vi "Execute.LoadSequences.vi"(8 "error in (no error)":errorcluster, 11 "Cluster":T1) -> (0 "error out":errorcluster)   [LabVIEW 2013, in "Simple Sequence Editor.lvlib"]
uses:
  Simple Sequence Editor.lvlib
  Types/Execuction.StateVariables.ctl
  Program Files/National Instruments/LabVIEW 2013/examples/NI Veristand/API/Execution API/Sequences/Stimulus Profile Control Tool/Project Execution State.ctl
  <vilib>/NI Veristand/Execution/DataLogging/DataLoggingSpecification Ref.ctl
  NationalInstruments.VeriStand.ClientAPI
  <vilib>/NI Veristand/Execution/DataLogging/IDataLogging Ref.ctl
  <vilib>/NI Veristand/Execution/Workspace/WorkspaceAPI.ctl
  NationalInstruments.VeriStand.RealTimeSequenceDefinitionApi
  Types/Execute.UserEventRefs.ctl
  <vilib>/NI Veristand/Execution/Workspace/SystemStateRegEventRef.ctl
  <vilib>/NI Veristand/Execution/Workspace/SystemStateEventRef.ctl
  NationalInstruments.VeriStand.Internal
  <vilib>/NI Veristand/Execution/Workspace/NI_VS Workspace ExecutionAPI.lvlib
  <vilib>/NI Veristand/Execution/DataLogging/NI_VS Data Logging API.lvlib
panel:
  out "Channels":string[](array[string])
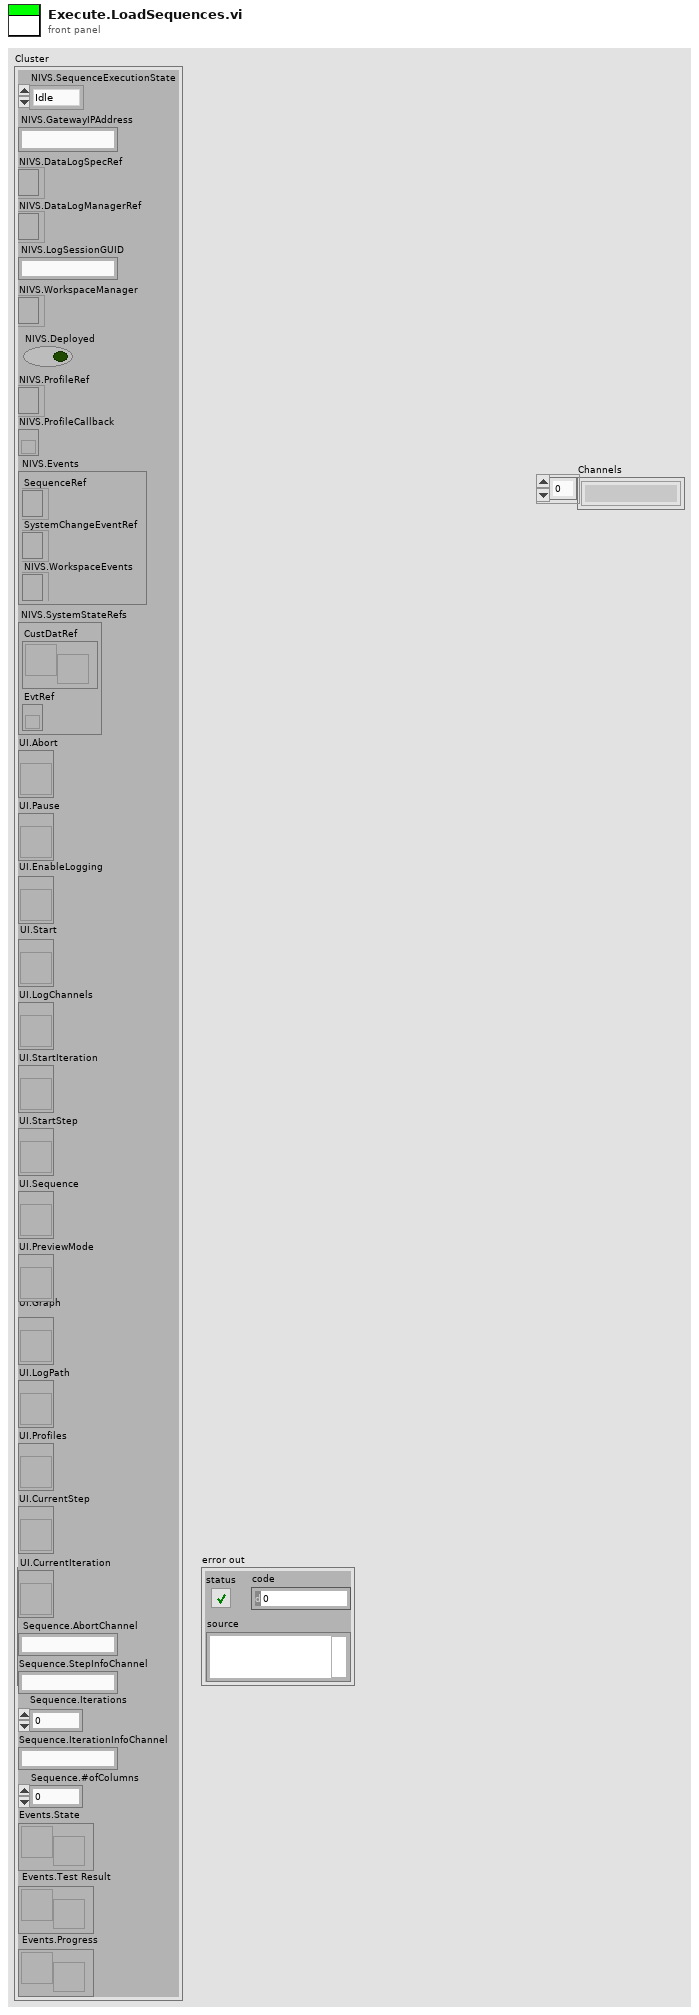
[diagram p1: front panel]
types:
  T1 = typedef "Simple Sequence Editor.lvlib/Execuction.StateVariables.ctl" = cluster{"NIVS.SequenceExecutionState":T2, "NIVS.GatewayIPAddress":string, "NIVS.DataLogSpecRef":T3, "NIVS.DataLogManagerRef":T4, "NIVS.LogSessionGUID":string, "NIVS.WorkspaceManager":T5, "NIVS.Deployed":bool, "NIVS.ProfileRef":refnum<k24>, "NIVS.ProfileCallback":refnum<k27>, "NIVS.Events":T6, "NIVS.SystemStateRefs":T8, "UI.Abort":refnum<vi>, "UI.Pause":refnum<vi>, "UI.EnableLogging":refnum<vi>, "UI.Start":refnum<vi>, "UI.LogChannels":refnum<vi>, "UI.StartIteration":refnum<vi>, "UI.StartStep":refnum<vi>, "UI.Sequence":refnum<vi>, "UI.PreviewMode":refnum<vi>, "UI.Graph":refnum<vi>, "UI.LogPath":refnum<vi>, "UI.Profiles":refnum<vi>, "UI.CurrentStep":refnum<vi>, "UI.CurrentIteration":refnum<vi>, "Sequence.AbortChannel":string, "Sequence.StepInfoChannel":string, "Sequence.Iterations":u32, "Sequence.IterationInfoChannel":string, "Sequence.#ofColumns":i32, "Events.State":refnum<user-event>, "Events.Test Result":refnum<user-event>, "Events.Progress":refnum<user-event>}
  T2 = typedef "Project Execution State.ctl" = enum16{"Idle", "Initializing", "Running", "Paused", "Finalizing", "Complete"}
  T3 = typedef "NI_VS Data Logging API.lvlib/DataLoggingSpecification Ref.ctl" = refnum<k24>
  T4 = typedef "NI_VS Data Logging API.lvlib/IDataLogging Ref.ctl" = refnum<k24>
  T5 = typedef "NI_VS Workspace ExecutionAPI.lvlib/WorkspaceAPI.ctl" = refnum<k24>
  T6 = typedef "Execute.UserEventRefs.ctl" = cluster{"SequenceRef":refnum<event-registration>, "SystemChangeEventRef":T7, "NIVS.WorkspaceEvents":refnum<event-registration>}
  T7 = typedef "NI_VS Workspace ExecutionAPI.lvlib/SystemStateRegEventRef.ctl" = refnum<event-registration>
  T8 = typedef "NI_VS Workspace ExecutionAPI.lvlib/SystemStateEventRef.ctl" = cluster{"CustDatRef":refnum<user-event>, "EvtRef":refnum<k27>}
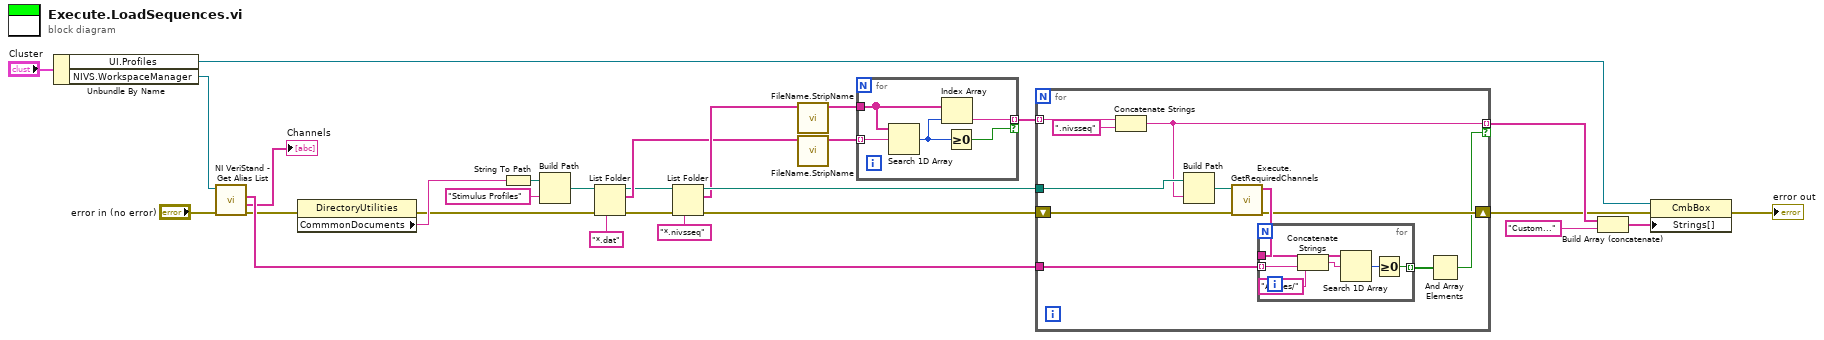
[diagram p0: block diagram]
diagram:
  n1 = Unbundle By Name("Cluster") -> ("UI.Profiles"=w23:refnum<vi>, "NIVS.WorkspaceManager"=w20:T5)
  n2 = call <vilib>:"NI VeriStand - Get Alias List.vi"("error in (no error)"="error in (no error)", "WorkspaceManager in"=w20) -> ("error out"=w4:errorcluster, "Channels"=→"Channels":string[], "Aliases"=w19:string[])  [unwired: 6 in, 1 out]
  n3 = property class="DirectoryUtilities"(error in=w4) -> (error out=w3:errorcluster, "CommmonDocuments"=w6:string)  [unwired: 1 in, 1 out]
  n4 = String To Path(string=w6) -> (path=w7:path)
  n5 = Build Path(base path=w7, name or relative path="Stimulus Profiles") -> (appended path=w2:path)
  n6 = List Folder(path=w2, pattern="*.dat", error in=w3) -> (path out=w8:path, filenames=w11:string[], error out=w16:errorcluster)  [unwired: 1 in, 1 out]
  n7 = List Folder(path=w8, pattern="*.nivsseq", error in=w16) -> (path out=w17:path, filenames=w13:string[], error out=w18:errorcluster)  [unwired: 1 in, 1 out]
  n8 = call "FileName.StripName.vi"("filenames"=w13) -> ("Array"=w14:string[])  [unwired: 10 in]
  n9 = call "FileName.StripName.vi"("filenames"=w11) -> ("Array"=w12:string[])  [unwired: 10 in]
  n10 = for {
    tunnel: w12 -> [w33] mode=indexing
    tunnel: w14 -> [w32]
    tunnel: [w30] -> w15 mode=indexing if=w29
    n11 = Search 1D Array(1D array=w32, element=w33) -> (index of element=w31:i32)  [unwired: 1 in]
    n12 = Index Array(array=w32, index=w31) -> (element=w30:string)
    n13 = Greater Or Equal To 0?(x=w31) -> (x >= 0?=w29:bool)
  }
  n14 = for {
    tunnel: w15 -> [w44] mode=indexing
    tunnel: w17 -> [w42]
    shift-right: [w36] -> w22
    shift-left: w18 -> [w41]
    tunnel: w19 -> [w38]
    tunnel: [w35] -> w24 mode=indexing if=w34
    n15 = Concatenate Strings(w44, ".nivsseq" ("pattern")) -> (w35:string)
    n16 = Build Path(base path=w42, name or relative path=w35) -> (appended path=w40:path)
    n17 = call "Execute.GetRequiredChannels.vi"("error in (no error)"=w41, "Path"=w40) -> ("error out"=w36:errorcluster, "Channels"=w39:string[])  [unwired: 8 in]
    n18 = for {
      tunnel: w39 -> [w50]
      tunnel: w38 -> [w49] mode=indexing
      tunnel: [w47] -> w37 mode=indexing
      n19 = Concatenate Strings("Aliases/", w49) -> (w46:string)
      n20 = Search 1D Array(1D array=w50, element=w46) -> (index of element=w48:i32)  [unwired: 1 in]
      n21 = Greater Or Equal To 0?(x=w48) -> (x >= 0?=w47:bool)
    }
    n22 = And Array Elements(Boolean array=w37) -> (logical AND=w34:bool)
  }
  n23 = Build Array (concatenate)(w24, "Custom...") -> (w25:string[])
  n24 = property class="CmbBox"(reference=w23, error in=w22, "Strings[]"=w25) -> (error out=→"error out":errorcluster)  [unwired: 1 out]
